vi "LightFieldFileNaming.vi"(4 "Cycle time\n(ms)":i32=3 min=0 step=1, 5 "On CCD Acc.":i32=3 min=0 step=1, 6 "Script#":i32, 7 "BG":bool, 8 "error in":errorcluster, 9 "BIN":u16(ring) items=["1x1", "2x2", "4x4"], 10 "MODE":u16(ring) items=["Normal", "DIF"], 11 "LightField Automation in":refnum<class "LightField Automation.lvclass">) -> (0 "error out":errorcluster, 3 "LightField Automation out":refnum<class "LightField Automation.lvclass">)   [LabVIEW 2018]
uses:
  LightField Automation.lvclass
  C:/Users/xw9/Desktop/Turbulence program/SourceDistribution/PrincetonInstruments.LightFieldAddInSupportServices.dll
  PrincetonInstruments.LightFieldAddInSupportServices.dll
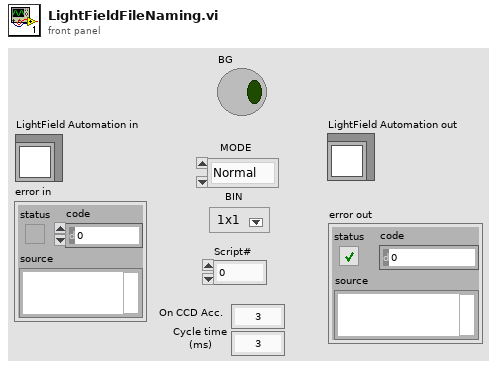
[diagram p1: front panel]
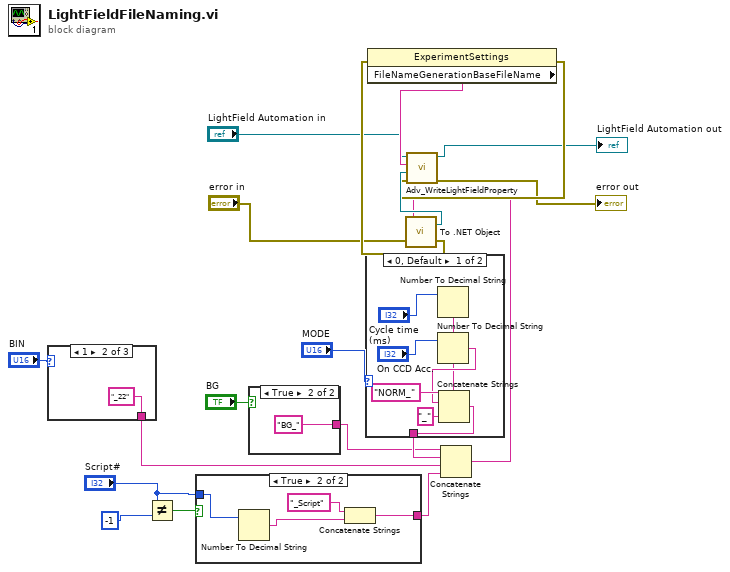
[diagram p0: block diagram]
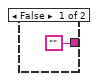
[diagram p2: hidden frame]
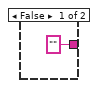
[diagram p3: hidden frame]
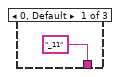
[diagram p4: hidden frame]
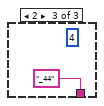
[diagram p5: hidden frame]
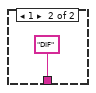
[diagram p6: hidden frame]
diagram:
  n1 = case shown="1" "BIN" {
    tunnel: ["_11" "_22" "_44"] -> w11
    frame 0, Default {
    }
    frame 1 {
    }
    frame 2 {
      (unwired) 4
    }
  }
  n2 = Not Equal?(x="Script#", y=-1) -> (x != y?=w9:bool)
  n3 = case shown="True" w9 {
    tunnel: "Script#" -> [_ w27]
    tunnel: ["" w24] -> w6
    frame False {
    }
    frame True {
      n4 = Number To Decimal String(number=w27) -> (decimal integer string=w25:string)  [unwired: 1 in]
      n5 = Concatenate Strings("_Script" ("string"), w25) -> (w24:string)
    }
  }
  n6 = case shown="True" "BG" {
    tunnel: ["" "BG_"] -> w2
    frame False {
    }
    frame True {
    }
  }
  n7 = case shown="0, Default" "MODE" {
    tunnel: [w34 "DIF"] -> w12
    frame 0, Default {
      n8 = Number To Decimal String(number="Cycle time\n(ms)") -> (decimal integer string=w30:string)  [unwired: 1 in]
      n9 = Number To Decimal String(number="On CCD Acc.") -> (decimal integer string=w31:string)  [unwired: 1 in]
      n10 = Concatenate Strings("NORM_", w31, "_" ("string"), w30) -> (w34:string)
    }
    frame 1 {
    }
  }
  n11 = Concatenate Strings(w2, w12, w11, w6) -> (w10:string)
  n12 = call "To .NET Object.vi"("error in (no error)"="error in", "anything"=w10) -> ("error out"=w15:errorcluster, ".NET object"=w17:refnum<k24>)
  n13 = property class="ExperimentSettings"(error in=w15) -> (error out=w16:errorcluster, "FileNameGenerationBaseFileName"=w18:string)  [unwired: 1 in, 1 out]
  n14 = call "Adv_WriteLightFieldProperty.vi"("error in (no error)"=w16, "value"=w17, "setting"=w18, "LightField Automation in"="LightField Automation in") -> ("error out"=→"error out":errorcluster, "LightField Automation out"=→"LightField Automation out":refnum<class "LightField Automation.lvclass">)  [unwired: 6 in]
